vi "Sequence.GenerateSequence.vi"(7 "Exists":bool, 8 "error in (no error)":errorcluster, 10 "Compiled Settings":T1, 11 "Path":path) -> (0 "error out":errorcluster)   [LabVIEW 2015, in "Single Station Execution.lvlib"]
uses:
  Single Station Execution.lvlib
  Types/Compiled.RTSequenceProperties.ctl
  Types/Channel.Properties.ctl
  Types/Compiled.StepProperties.ctl
  Types/Compiled.IOStateProperties.ctl
  Types/Compiled.StepElementProperties.ctl
  Types/Step.Types.ctl
  Types/Compiled.StepCondition.ctl
  Types/Conditions.OperationTypes.ctl
  Types/Compiled.SequenceChannels.ctl
  NationalInstruments.VeriStand.RealTimeSequenceDefinitionApi
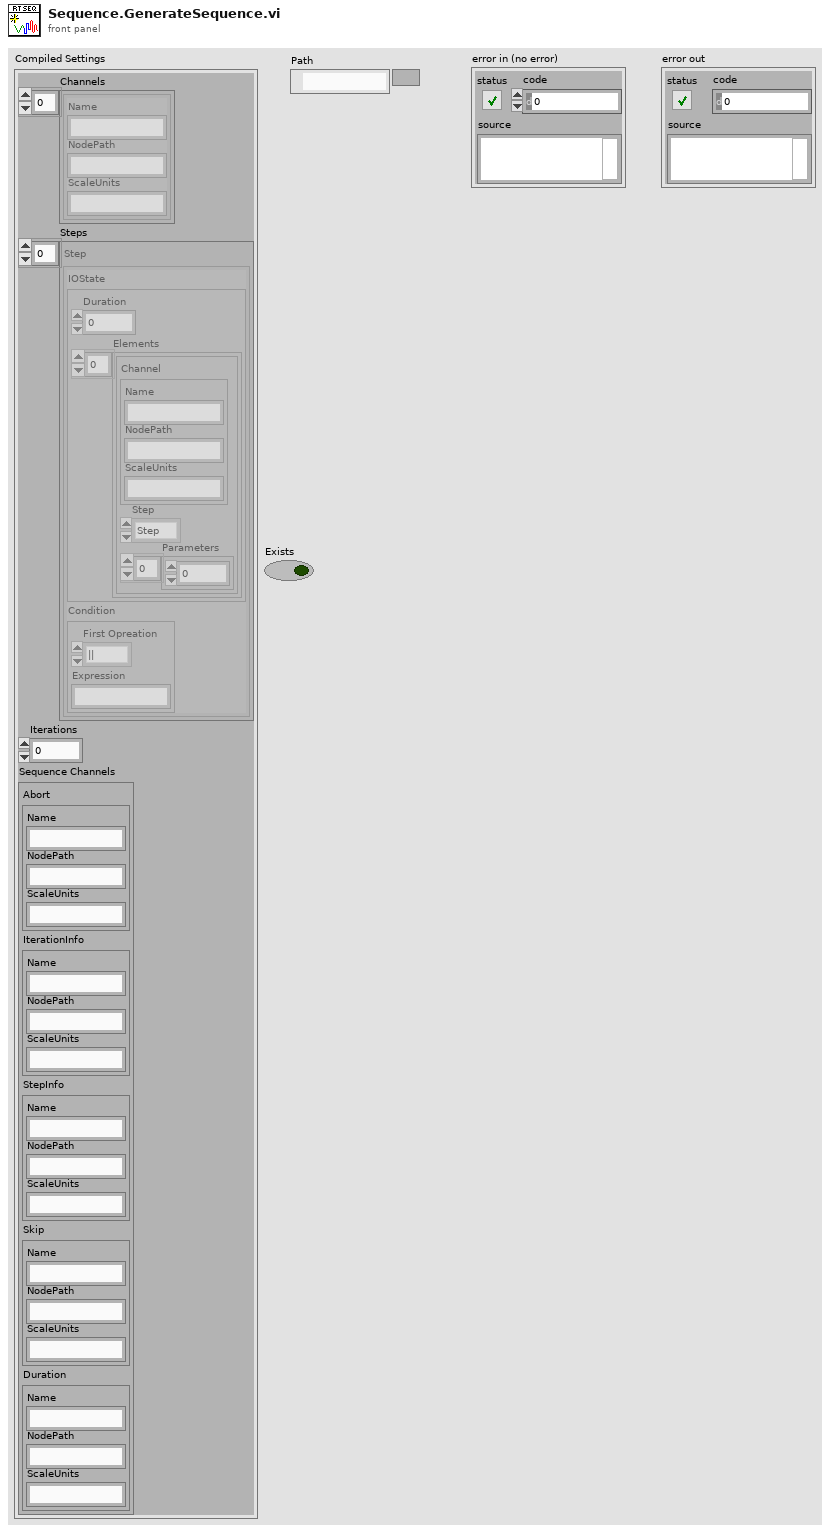
[diagram p1: front panel]
types:
  T1 = typedef "Single Station Execution.lvlib/Compiled.RTSequenceProperties.ctl" = cluster{"Channels":T2[], "Steps":T3[], "Iterations":u32, "Sequence Channels":T9}
  T2 = typedef "Single Station Execution.lvlib/Channel.Properties.ctl" = cluster{"Name":string, "NodePath":string, "ScaleUnits":string}
  T3 = typedef "Single Station Execution.lvlib/Compiled.StepProperties.ctl" = cluster{"IOState":T4, "Condition":T7}
  T4 = typedef "Single Station Execution.lvlib/Compiled.IOStateProperties.ctl" = cluster{"Duration":dbl, "Elements":T5[]}
  T5 = typedef "Single Station Execution.lvlib/Compiled.StepElementProperties.ctl" = cluster{"Channel":T2, "Step":T6, "Parameters":dbl[]}
  T6 = typedef "Single Station Execution.lvlib/Step.Types.ctl" = enum8{"Step", "iStep", "Ramp", "Unchanged", "Unknown", "Sine", "LogSine", "LinearSine", "ForcedRamp", "Waveform"}
  T7 = typedef "Single Station Execution.lvlib/Compiled.StepCondition.ctl" = cluster{"First Opreation":T8, "Expression":string}
  T8 = typedef "Single Station Execution.lvlib/Conditions.OperationTypes.ctl" = enum8{"None", "&&", "||"}
  T9 = typedef "Single Station Execution.lvlib/Compiled.SequenceChannels.ctl" = cluster{"Abort":T2, "IterationInfo":T2, "StepInfo":T2, "Skip":T2, "Duration":T2}
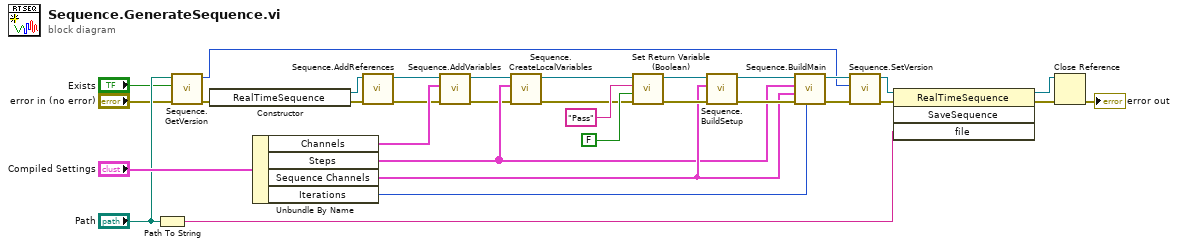
[diagram p0: block diagram]
diagram:
  n1 = Path To String(path="Path") -> (string=w25:string)
  n2 = call "Sequence.GetVersion.vi"("error in (no error)"="error in (no error)", "Exists"="Exists", "Path"="Path") -> ("error out"=w12:errorcluster, "Build"=w6:u32)  [unwired: 7 in]
  n3 = constructor class="RealTimeSequence"(error in=w12) -> (reference out=w24:refnum<k24>, error out=w17:errorcluster)  [unwired: 2 in, 1 out]
  n4 = Unbundle By Name("Compiled Settings") -> ("Channels"=w28:T2[], "Steps"=w5:T3[], "Sequence Channels"=w15:T9, "Iterations"=w16:u32)
  n5 = call "Sequence.AddReferences.vi"("error in (no error)"=w17, "Sequence"=w24) -> ("error out"=w22:errorcluster, "Sequence out"=w23:refnum<k24>)  [unwired: 8 in]
  n6 = call "Sequence.AddVariables.vi"("error in (no error)"=w22, "Channels"=w28, "Sequence"=w23) -> ("error out"=w4:errorcluster, "Sequence out"=w2:refnum<k24>)  [unwired: 7 in]
  n7 = call "Sequence.CreateLocalVariables.vi"("error in (no error)"=w4, "Steps"=w5, "Sequence Ref"=w2) -> ("error out"=w3:errorcluster, "Sequence Ref out"=w1:refnum<k24>)  [unwired: 7 in]
  n8 = call "Set Return Variable (Boolean).vi"("error in (no error)"=w3, "Value"=FALSE, "Identifier"="Pass", "Sequence Ref in"=w1) -> ("error out"=w21:errorcluster, "Sequence Ref out"=w20:refnum<k24>)  [unwired: 6 in]
  n9 = call "Sequence.BuildSetup.vi"("error in (no error)"=w21, "Sequence Channels"=w15, "Sequence"=w20) -> ("error out"=w18:errorcluster, "Sequence out"=w19:refnum<k24>)  [unwired: 7 in]
  n10 = call "Sequence.BuildMain.vi"("Iterations"=w16, "error in (no error)"=w18, "Sequence Channels"=w15, "Steps"=w5, "Sequence"=w19) -> ("error out"=w10:errorcluster, "Sequence out"=w8:refnum<k24>)  [unwired: 5 in]
  n11 = call "Sequence.SetVersion.vi"("error in (no error)"=w10, "BuildVersion"=w6, "RT Seq Ref"=w8) -> ("error out"=w9:errorcluster, "RT Seq Ref out"=w7:refnum<k24>)  [unwired: 7 in]
  n12 = invoke class="RealTimeSequence" method="SaveSequence"(reference=w7, error in=w9, "file"=w25) -> (reference out=w32:refnum<k24>, error out=w27:errorcluster)  [unwired: 1 in, 2 out]
  n13 = Close Reference(reference=w32, error in (no error)=w27) -> (error out=→"error out":errorcluster)
